vi "Call Main VI.vi"   [LabVIEW 2010]
uses:
  Source Code/SubVIs/User Login Relative.llb/Login Info__BMA-ULR.ctl
types:
  T1 = typedef "Login Info__BMA-ULR.ctl" = cluster{"status":bool, "account":u16, "user":string}
  T2 = typedef "Path InitDynamicVIsPaths__FS.ctl" = cluster{"F4 Operation":path, "F4 Alarms":path, "F4 Inputs":path, "F4 Outputs":path, "F4 PID Sets":path, "F4 Cascade":path, "F4 Current Step":path, "Profile SubPanel":path, "Profile Editor":path, "MainVI":path, "Profile Control":path, "Synergy Control":path, "Driver Server":path}
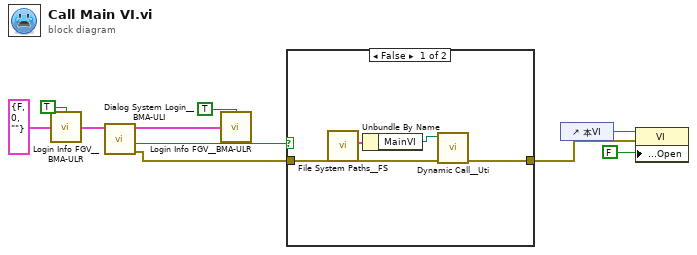
[diagram p0: block diagram]
diagram:
  n1 = call "Login Info FGV__BMA-ULR.vi"("login info in"=T1 {"status"=FALSE, "account"=0, "user"=""}, "read/write (F:read)"=TRUE) -> ("login info out"=w9:T1)
  n2 = call "Dialog System Login__BMA-ULI.vi"("login info in"=w9) -> ("error out"=w4:errorcluster, "failed at first login?"=w7:bool, "login info out"=w8:T1)  [unwired: 8 in]
  n3 = call "Login Info FGV__BMA-ULR.vi"("login info in"=w8, "read/write (F:read)"=TRUE) -> ()  [unwired: 1 out]
  n4 = case shown="False" w7 {
    tunnel: [w12 w16] -> w5
    tunnel: w4 -> [w11 w16]
    frame False {
      n5 = call "File System Paths__FS.vi"("error in (no error)"=w11) -> ("error out"=w13:errorcluster, "DynamicVIs"=w15:T2)  [unwired: 8 in, 1 out]
      n6 = Unbundle By Name(w15) -> ("MainVI"=w14:path)
      n7 = call "Dynamic Call__Uti.vi"("error in (no error)"=w13, "vi path"=w14) -> ("error out"=w12:errorcluster)  [unwired: 9 in]
    }
    frame True {
    }
  }
  n8 = control-ref of="本VI"() -> (w6:refnum<vi>)
  n9 = property class="VI"(reference=w6, error in=w5, "Front Panel.Open"=FALSE ("前面板窗口:打开")) -> ()  [unwired: 2 out]
